vi "seq_to_var_string.vi"(11 "SEQs IN":T1[](array[typedef])) -> (0 "VAR Strings":string[](array[string]), 3 "SEQs OUT":T1[](array[typedef]))   [LabVIEW 2015, in "oskar_tools.lvlib"]
uses:
  oskar_tools.lvlib
  seq_line.ctl
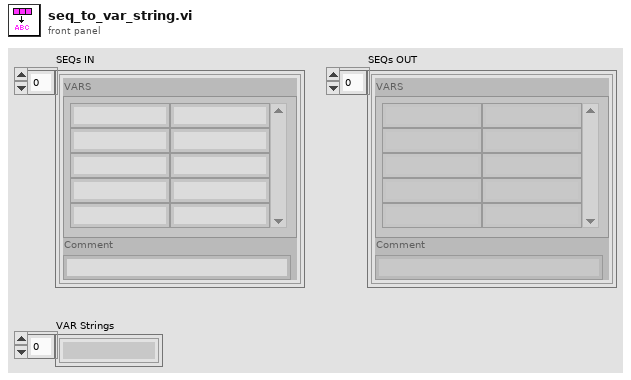
[diagram p1: front panel]
types:
  T1 = typedef "oskar_tools.lvlib/seq_line.ctl" = cluster{"VARS":string[][], "Comment":string}
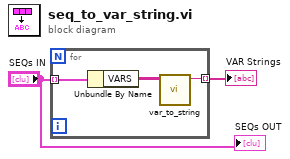
[diagram p0: block diagram]
diagram:
  n1 = for {
    tunnel: "SEQs IN" -> [w5] mode=indexing
    tunnel: [w3] -> w1 mode=indexing
    n2 = Unbundle By Name(w5) -> ("VARS"=w4:string[][])
    n3 = call "var_to_string.vi"("Var Array"=w4) -> ("VAR string"=w3:string)  [unwired: 10 in]
  }
  "VAR Strings" <- w1
  "SEQs OUT" <- "SEQs IN"
